vi "Color Sensor Global.vi"() -> ()   [LabVIEW 2019]
panel:
  in  "Color":dbl
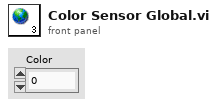
[diagram p1: front panel]
diagram:
